vi "Sub_Read_MQTT_String.vi"(8 "error in (no error)":errorcluster, 10 "UTF8 Byte Array":u8[](array[numeric]) format="%x") -> (0 "error out":errorcluster, 1 "remaining bytes":u8[](array[numeric]) format="%x", 2 "String":string="MQIsdp")   [LabVIEW 2018, in "MQTT_Functions.lvlib"]
uses:
  MQTT_Functions.lvlib
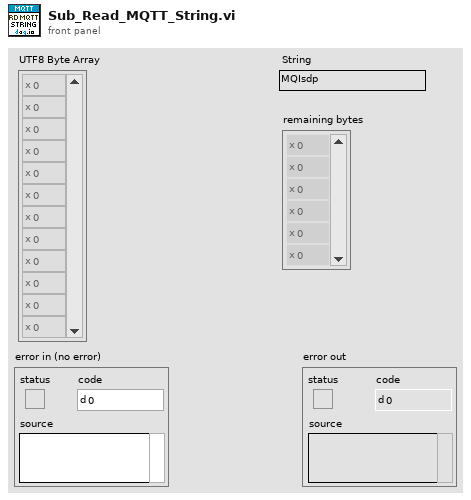
[diagram p1: front panel]
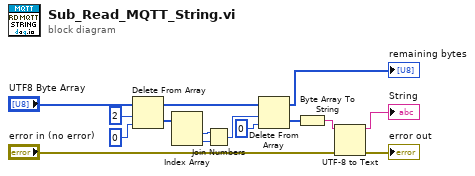
[diagram p0: block diagram]
diagram:
  n1 = Delete From Array(array="UTF8 Byte Array", length=2, index=0) -> (deleted portion=w4:u8[], array with subset deleted=w5:u8[])
  n2 = Index Array(array=w4) -> (element #1=w7:u8, element #2=w6:u8)  [unwired: 2 in]
  n3 = Join Numbers(hi=w7, lo=w6) -> ((hi.lo)=w11:u16)
  n4 = Delete From Array(array=w5, length=w11, index=0) -> (deleted portion=w3:u8[], array with subset deleted=→"remaining bytes":u8[])
  n5 = Byte Array To String(unsigned byte array=w3) -> (string=w14:string)
  n6 = UTF-8 to Text(8:"error in (no error)", 11:w14) -> (0:→"error out":errorcluster, 3:→"String":string)  [unwired: 1 in]
